vi "Main.vi"() -> ()   [LabVIEW 2019]
uses:
  UI/Channel Controls.ctl
  UI/Channel Control.ctl
  Controller/Serial Info.ctl
  UI/UI State.ctl
  UI/Update Message.ctl
  UI/Update Command.ctl
  Controller/Controller Message.ctl
  Controller/MDS Command.ctl
  UI/UI.lvlib
  Controller/Controller.lvlib
  Listener/Listener.lvlib
panel:
  in  "Listener":T1={"Port"="", "Baud Rate"=19200} {"Baud Rate" format="%.0f bps"}
  in  "Controller B":T1={"Port"="", "Baud Rate"=19200} {"Baud Rate" format="%.0f bps"}
  in  "Controller A":T1={"Port"="", "Baud Rate"=19200} {"Baud Rate" format="%.0f bps"}
  in  "Emulate":bool
  in  "Int-Ext":bool caption="Emulate"
  in  "Quit":bool
  in  "Connect":bool caption="Emulate"
  in  "Channels":T2 {"Frequency" format="%#_g MHz"; "Power" format="%#_g dBm"}
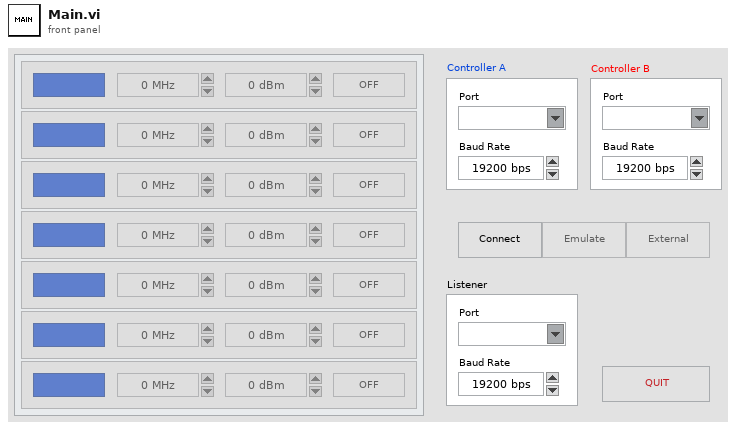
[diagram p1: front panel]
types:
  T1 = typedef "Controller.lvlib/Serial Info.ctl" = cluster{"Port":refnum<visa-resource-name>, "Baud Rate":u32}
  T2 = typedef "UI.lvlib/Channel Controls.ctl" = T3[]
  T3 = typedef "UI.lvlib/Channel Control.ctl" = cluster{"Power":dbl, "Frequency":dbl, "PLL":bool, "A/B":bool}
  T4 = typedef "UI.lvlib/UI State.ctl" = enum16{"Init", "Idle", "Update Buttons", "Connect", "Refresh Channels", "Disconnect", "Quit"}
  T5 = typedef "UI.lvlib/Main States.ctl" = cluster{"UI Queue":T6, "Controller A Queue":T7, "Controller B Queue":T7, "Listener Queue":T8}
  T6 = typedef "UI.lvlib/UI Message Queue.ctl" = refnum<queue>
  T7 = typedef "Controller.lvlib/Controller Message Queue.ctl" = refnum<queue>
  T8 = typedef "Listener.lvlib/Listener Message Queue.ctl" = refnum<queue>
  T9 = enum8{"Enabled", "Disabled", "Disabled and Grayed Out"}
  T10 = typedef "UI.lvlib/Update Message.ctl" = cluster{"Update Command":T11, "Channel":u8, "Value":variant}
  T11 = typedef "UI.lvlib/Update Command.ctl" = enum16{"Update Frequency", "Update Power", "Update Switch", "Error", "Stop"}
  T12 = typedef "Controller.lvlib/Controller Message.ctl" = cluster{"MDS Command":T13, "Channel":u8, "Value":variant}
  T13 = typedef "Controller.lvlib/MDS Command.ctl" = enum16{"Idle", "Open", "Set VMode", "Set IMode", "Get Frequency", "Set Frequency", "Get Power", "Set Power (dBm)", "Set Power (%)", "Get Switch", "Switch Channel", "Store", "Wait for Prompt", "Wait for State", "Reset", "Error", "Close", "Stop"}
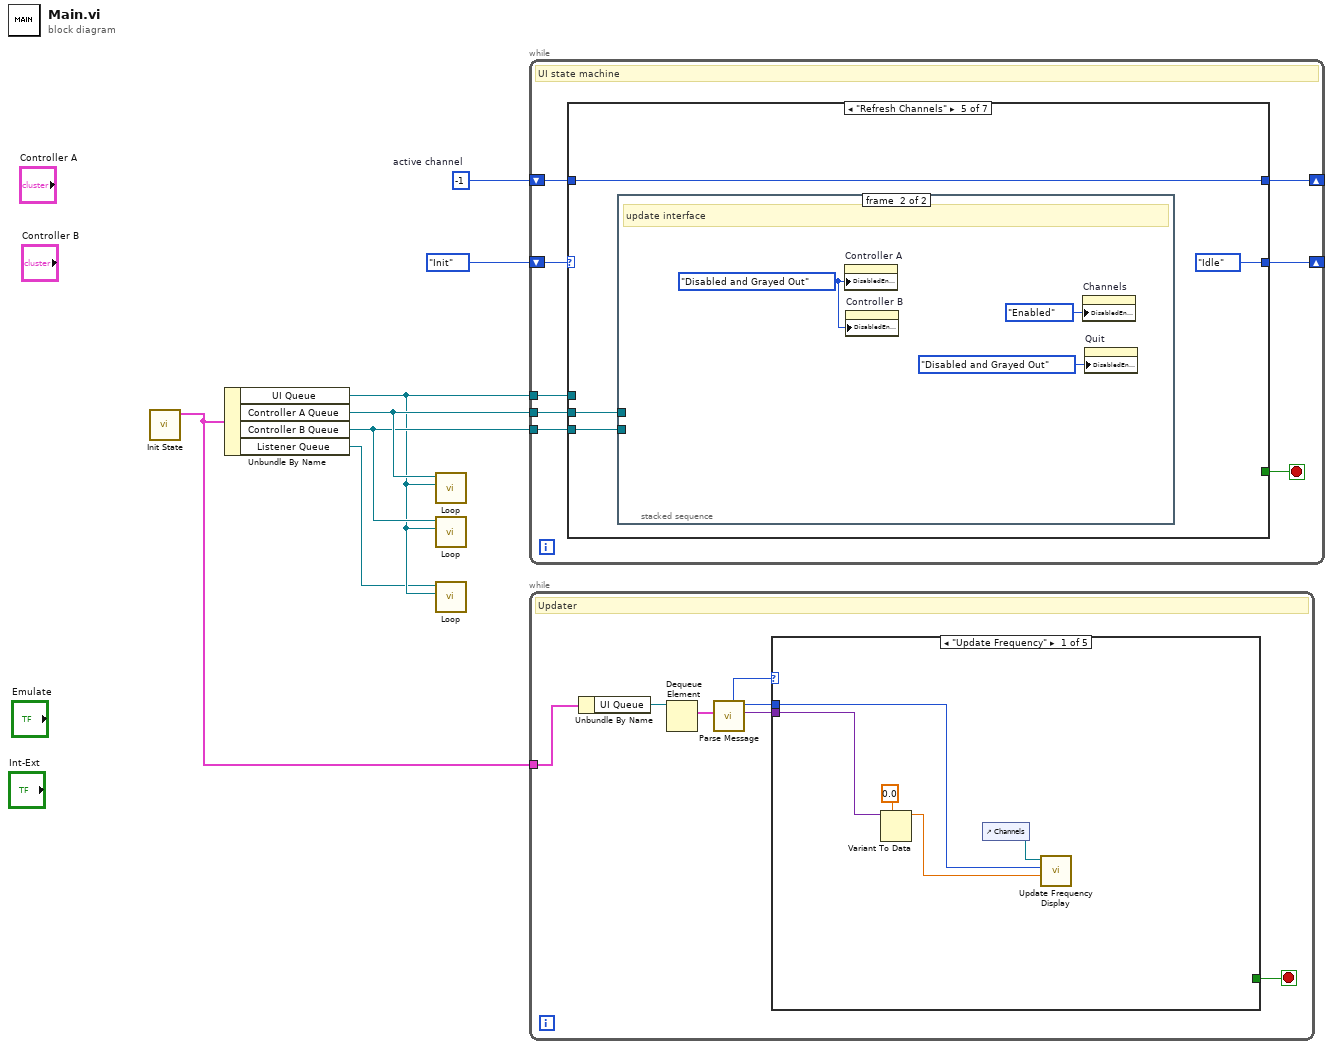
[diagram p0: block diagram]
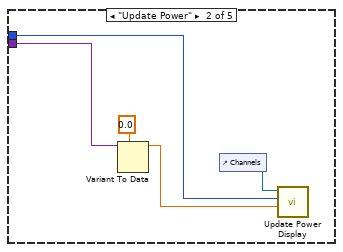
[diagram p2: hidden frame]
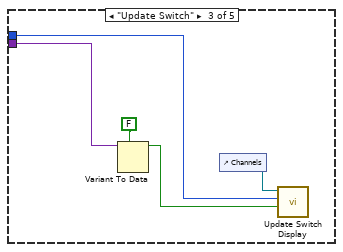
[diagram p3: hidden frame]
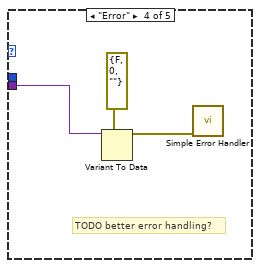
[diagram p4: hidden frame]
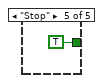
[diagram p5: hidden frame]
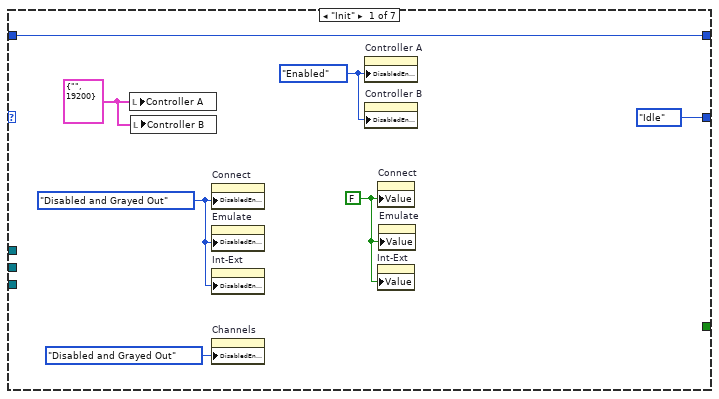
[diagram p6: hidden frame]
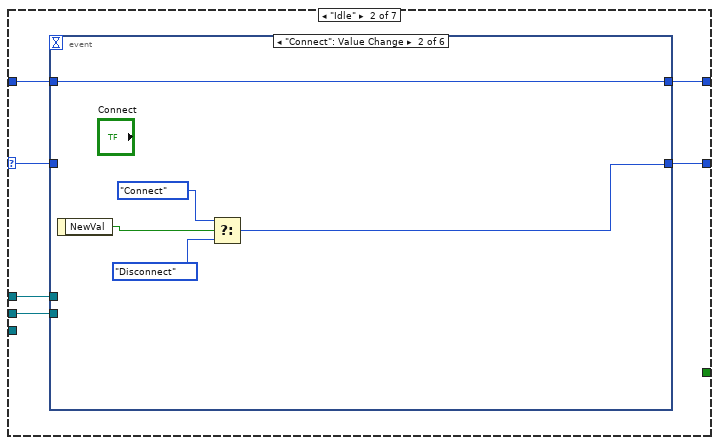
[diagram p7: hidden frame]
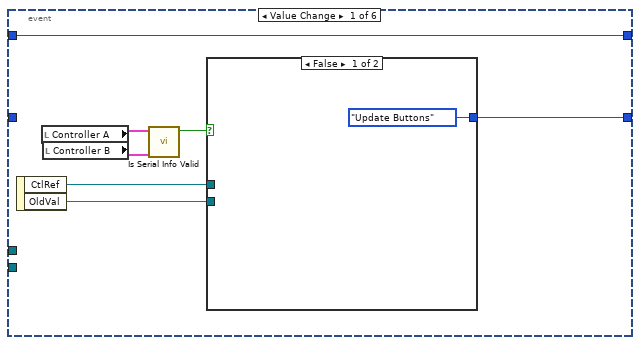
[diagram p8: hidden frame]
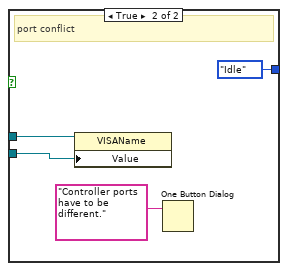
[diagram p9: hidden frame]
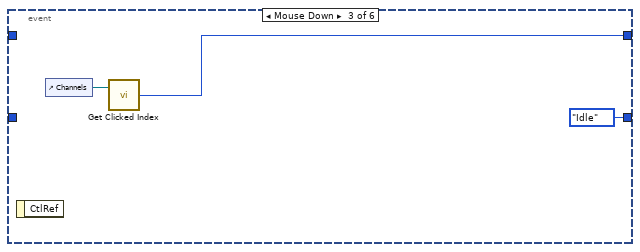
[diagram p10: hidden frame]
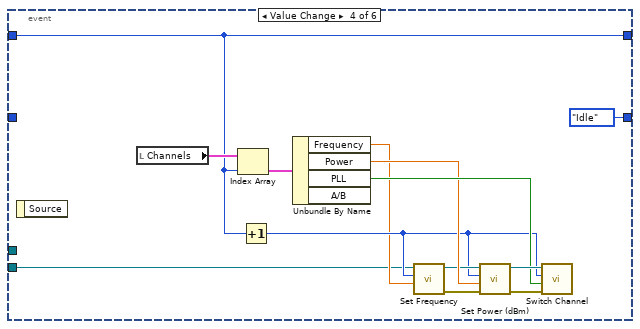
[diagram p11: hidden frame]
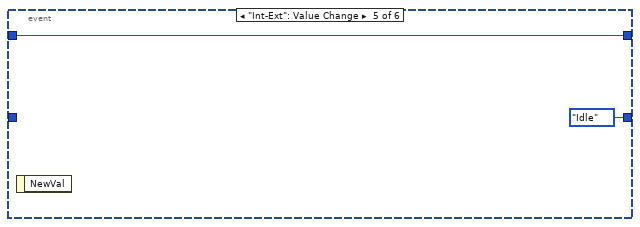
[diagram p12: hidden frame]
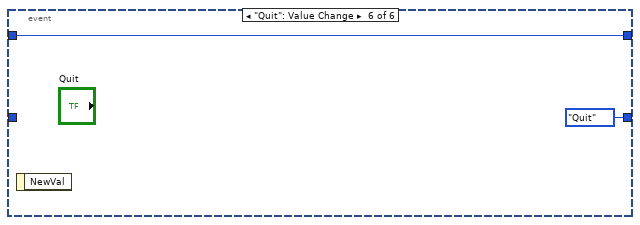
[diagram p13: hidden frame]
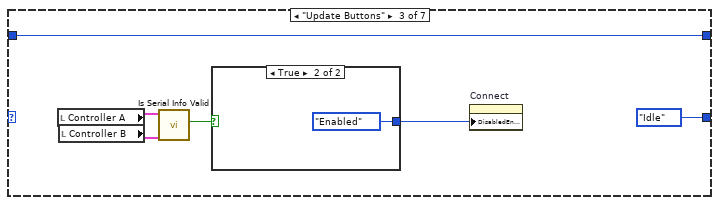
[diagram p14: hidden frame]
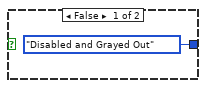
[diagram p15: hidden frame]
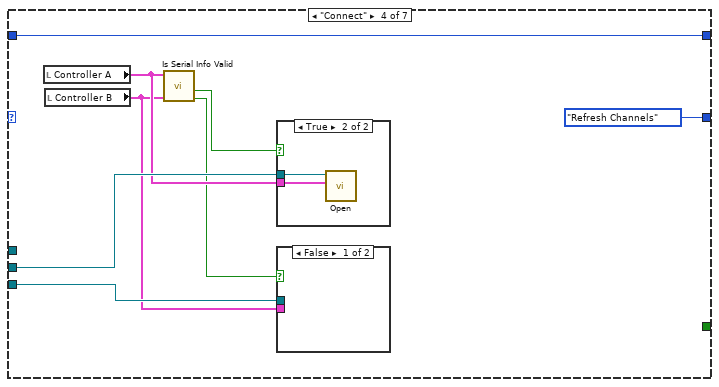
[diagram p16: hidden frame]
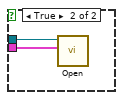
[diagram p17: hidden frame]
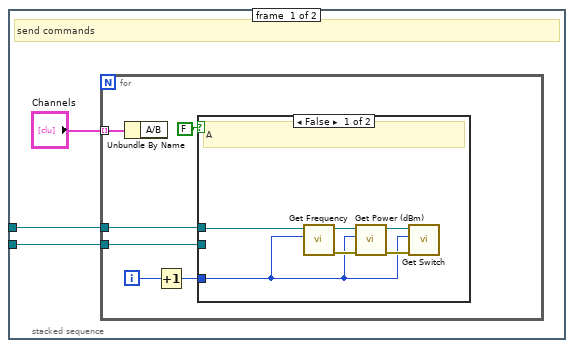
[diagram p19: hidden frame]
diagram:
  w4 = -1  # active channel
  n1 = call "Init State.vi"() -> ("Main State"=w7:T5)  [unwired: 11 in]
  n2 = Unbundle By Name(w7) -> ("UI Queue"=w2:T6, "Controller A Queue"=w5:T7, "Controller B Queue"=w3:T7, "Listener Queue"=w1:T8)
  n3 = call "Loop.vi"("UI Queue"=w2, "Controller Queue"=w5) -> ()  [unwired: 9 in, 1 out]
  n4 = call "Loop.vi"("UI Queue"=w2, "Controller Queue"=w3) -> ()  [unwired: 9 in, 1 out]
  n5 = call "Loop.vi"("UI Queue"=w2, "Listener Queue"=w1) -> ()  [unwired: 9 in, 1 out]
  n6 = while {
    tunnel: w2 -> [w15]
    shift-right: [w12] -> _
    shift-left: UI_State."Init" ("UI States") -> [w13]
    tunnel: w5 -> [w11]
    tunnel: w3 -> [w10]
    shift-right: [w9] -> _
    shift-left: w4 -> [w8]
    stop <- w14 stop-if-true
    # "UI state machine"
    n7 = case shown="\"Refresh Channels\"" w13 {
      selector: w13 -> [_ w26 _ _ _ _ _]
      tunnel: w15 -> [_ w28 _ _ _ _ w128]
      tunnel: [_ _ _ _ _ _ TRUE] -> w14
      tunnel: [UI_State."Idle" ("UI States") w27 UI_State."Idle" ("UI States") UI_State."Refresh Channels" ("UI States") UI_State."Idle" ("UI States") UI_State."Idle" ("UI States") UI_State."Quit" ("UI States")] -> w12
      tunnel: w11 -> [_ w25 _ w79 w88 w110 w126]
      tunnel: w10 -> [_ _ _ w76 w87 w109 w124]
      tunnel: [w16 w24 w66 w74 w86 w108 w125] -> w9
      tunnel: w8 -> [w16 w23 w66 w74 w86 w108 w125]
      frame "Init" {
        w17 = FALSE ("Connect")
        w18 = T9."Enabled" ("Disabled")
        w20 = T9."Disabled and Grayed Out" ("Disabled")
        w21 = T1 {"Port"="", "Baud Rate"=19200} ("Controller A")
        n8 = local write "Controller A"(w21) -> ()
        n9 = local write "Controller B"(w21) -> ()
        n10 = property on="Connect" class="Bool (strict)"("DisabledEnum"=w20) -> ()  [unwired: 2 in, 2 out]
        n11 = property on="Emulate" class="Bool (strict)"("DisabledEnum"=w20) -> ()  [unwired: 2 in, 2 out]
        n12 = property on="Int-Ext" class="Bool (strict)"("DisabledEnum"=w20) -> ()  [unwired: 2 in, 2 out]
        n13 = property on="Channels" class="Arr"("DisabledEnum"=T9."Disabled and Grayed Out" ("Disabled")) -> ()  [unwired: 2 in, 2 out]
        n14 = property on="Controller A" class="Clust (strict)"("DisabledEnum"=w18) -> ()  [unwired: 2 in, 2 out]
        n15 = property on="Controller B" class="Clust (strict)"("DisabledEnum"=w18) -> ()  [unwired: 2 in, 2 out]
        n16 = property on="Connect" class="Bool (strict)"("Value"=w17) -> ()  [unwired: 2 in, 2 out]
        n17 = property on="Int-Ext" class="Bool (strict)"("Value"=w17) -> ()  [unwired: 2 in, 2 out]
        n18 = property on="Emulate" class="Bool (strict)"("Value"=w17) -> ()  [unwired: 2 in, 2 out]
      }
      frame "Idle" {
        n19 = event shown="[1] \"Connect\": Value Change" {
          selector: _ -> [_ _ _ _ _ _]
          dyn-events: _ -> [_ _ _ _ _ _]
          timeout: _ -> [_ _ _ _ _ _]
          tunnel: w28 -> [_ _ _ _ _ _]
          tunnel: [w30 w43 UI_State."Idle" ("UI States") UI_State."Idle" ("UI States") UI_State."Idle" ("UI States") UI_State."Quit" ("UI States")] -> w27
          tunnel: w26 -> [_ _ _ _ _ _]
          tunnel: w25 -> [_ _ _ w51 _ _]
          tunnel: [w29 w41 w46 w50 w63 w64] -> w24
          tunnel: w23 -> [w29 w41 _ w50 w63 w64]
          event Value Change {
            n20 = event-data() -> ("CtlRef"=w34:refnum<vi>, "OldVal"=w33:refnum<visa-resource-name>)  [unwired: 1 in]
            n21 = local read "Controller A"() -> (w32:T1)
            n22 = local read "Controller B"() -> (w31:T1)
            n23 = call "Is Serial Info Valid.vi"("Controller B"=w31, "Controller A"=w32) -> ("Conflict?"=w35:bool)  [unwired: 6 in, 3 out]
            n24 = case shown="False" w35 {
              tunnel: w34 -> [_ w40]
              tunnel: w33 -> [_ w39]
              tunnel: [UI_State."Update Buttons" ("UI States") UI_State."Idle" ("UI States")] -> w30
              frame False {
              }
              frame True {
                # "port conflict"
                n25 = property class="VISAName"(reference=w40, "Value"=w39) -> ()  [unwired: 1 in, 2 out]
                n26 = One Button Dialog(message="Controller ports have to be different.") -> ()  [unwired: 1 in, 1 out]
              }
            }
          }
          event "Connect": Value Change {
            n27 = event-data() -> ("NewVal"=w45:bool)  [unwired: 1 in]
            n28 = Select(t=UI_State."Connect" ("UI States"), s=w45, f=UI_State."Disconnect") -> (s? t:f=w43:T4)
          }
          event Mouse Down {
            n29 = event-data() -> ()  [unwired: 1 in, 1 out]
            n30 = control-ref of="Channels"() -> (w47:refnum<vi>)
            n31 = call "Get Clicked Index.vi"("Refnum in"=w47) -> ("Index"=w46:u32)  [unwired: 1 in]
          }
          event Value Change {
            n32 = event-data() -> ()  [unwired: 1 in, 1 out]
            n33 = local read "Channels"() -> (w61:T2)
            n34 = Index Array(array=w61, index=w50) -> (element=w60:T3)
            n35 = Increment(x=w50) -> (x+1=w54:u32)
            n36 = Unbundle By Name(w60) -> ("Frequency"=w53:dbl, "Power"=w56:dbl, "PLL"=w57:bool)  [unwired: 1 out]
            n37 = call "Set Frequency.vi"("Frequency (MHz)"=w53, "Channel"=w54, "Queue in"=w51) -> ("error out"=w52:errorcluster, "Queue out"=w55:T7)  [unwired: 7 in]
            n38 = call "Set Power (dBm).vi"("error in (no error)"=w52, "Power (dBm)"=w56, "Channel"=w54, "Queue in"=w55) -> ("error out"=w58:errorcluster, "Queue out"=w59:T7)  [unwired: 6 in]
            n39 = call "Switch Channel.vi"("error in (no error)"=w58, "On/Off"=w57, "Channel"=w54, "Queue in"=w59) -> ()  [unwired: 6 in, 2 out]
          }
          event "Int-Ext": Value Change {
            n40 = event-data() -> ()  [unwired: 1 in, 1 out]
          }
          event "Quit": Value Change {
            n41 = event-data() -> ()  [unwired: 1 in, 1 out]
          }
        }
      }
      frame "Update Buttons" {
        n42 = local read "Controller A"() -> (w70:T1)
        n43 = local read "Controller B"() -> (w69:T1)
        n44 = call "Is Serial Info Valid.vi"("Controller B"=w69, "Controller A"=w70) -> ("Has Valid?"=w68:bool)  [unwired: 6 in, 3 out]
        n45 = case shown="True" w68 {
          tunnel: [T9."Disabled and Grayed Out" ("Disabled") T9."Enabled" ("Disabled")] -> w67
          frame False {
          }
          frame True {
          }
        }
        n46 = property on="Connect" class="Bool (strict)"("DisabledEnum"=w67) -> ()  [unwired: 2 in, 2 out]
      }
      frame "Connect" {
        n47 = local read "Controller A"() -> (w78:T1)
        n48 = local read "Controller B"() -> (w75:T1)
        n49 = call "Is Serial Info Valid.vi"("Controller B"=w75, "Controller A"=w78) -> ("B Valid?"=w77:bool, "A Valid?"=w80:bool)  [unwired: 6 in, 2 out]
        n50 = case shown="True" w80 {
          tunnel: w79 -> [_ w85]
          tunnel: w78 -> [_ w84]
          frame False {
          }
          frame True {
            n51 = call "Open.vi"("Serial Info"=w84, "Controller Queue in"=w85) -> ()  [unwired: 8 in, 2 out]
          }
        }
        n52 = case shown="False" w77 {
          tunnel: w76 -> [_ w83]
          tunnel: w75 -> [_ w82]
          frame False {
          }
          frame True {
            n53 = call "Open.vi"("Serial Info"=w82, "Controller Queue in"=w83) -> ()  [unwired: 8 in, 2 out]
          }
        }
      }
      frame "Refresh Channels" {
        n54 = stacked-sequence {
          tunnel: w88 -> [w91 _]
          tunnel: w87 -> [w90 _]
          frame #0 {
            # "send commands"
            n55 = for {
              tunnel: "Channels" -> [w98] mode=indexing
              tunnel: w91 -> [w96]
              tunnel: w90 -> [w95]
              i -> [w94]
              n56 = Unbundle By Name(w98) -> ()  [unwired: 1 out]
              n57 = Increment(x=w94) -> (x+1=w93:i32)
              n58 = case shown="False" FALSE {
                tunnel: w96 -> [w104 _]
                tunnel: w95 -> [_ _]
                tunnel: w93 -> [w99 _]
                frame False {
                  # "A"
                  n59 = call "Get Frequency.vi"("Channel"=w99, "Queue in"=w104) -> ("error out"=w102:errorcluster, "Queue out"=w103:T7)  [unwired: 8 in]
                  n60 = call "Get Power (dBm).vi"("error in (no error)"=w102, "Channel"=w99, "Queue in"=w103) -> ("error out"=w100:errorcluster, "Queue out"=w101:T7)  [unwired: 7 in]
                  n61 = call "Get Switch.vi"("error in (no error)"=w100, "Channel"=w99, "Queue in"=w101) -> ()  [unwired: 7 in, 2 out]
                }
                frame True {
                  # "B"
                }
              }
            }
          }
          frame #1 {
            w105 = T9."Disabled and Grayed Out" ("Disabled")
            # "update interface"
            n62 = property on="Controller A" class="Clust (strict)"("DisabledEnum"=w105) -> ()  [unwired: 2 in, 2 out]
            n63 = property on="Controller B" class="Clust (strict)"("DisabledEnum"=w105) -> ()  [unwired: 2 in, 2 out]
            n64 = property on="Channels" class="Arr"("DisabledEnum"=T9."Enabled" ("Disabled")) -> ()  [unwired: 2 in, 2 out]
            n65 = property on="Quit" class="Bool"("DisabledEnum"=T9."Disabled and Grayed Out" ("Disabled")) -> ()  [unwired: 2 in, 2 out]
          }
        }
      }
      frame "Disconnect" {
        n66 = stacked-sequence {
          tunnel: w110 -> [w116 _]
          tunnel: w109 -> [w113 _]
          frame #0 {
            # "send command"
            n67 = local read "Controller A"() -> (w115:T1)
            n68 = local read "Controller B"() -> (w112:T1)
            n69 = call "Is Serial Info Valid.vi"("Controller B"=w112, "Controller A"=w115) -> ("B Valid?"=w114:bool, "A Valid?"=w117:bool)  [unwired: 6 in, 2 out]
            n70 = case shown="True" w117 {
              tunnel: w116 -> [_ w119]
              frame False {
              }
              frame True {
                n71 = call "Close.vi"("Controller Queue in"=w119) -> ()  [unwired: 9 in, 2 out]
              }
            }
            n72 = case shown="False" w114 {
              tunnel: w113 -> [_ w118]
              frame False {
              }
              frame True {
                n73 = call "Close.vi"("Controller Queue in"=w118) -> ()  [unwired: 9 in, 2 out]
              }
            }
          }
          frame #1 {
            w120 = T9."Enabled" ("Disabled")
            # "update interface"
            n74 = property on="Controller A" class="Clust (strict)"("DisabledEnum"=w120) -> ()  [unwired: 2 in, 2 out]
            n75 = property on="Controller B" class="Clust (strict)"("DisabledEnum"=w120) -> ()  [unwired: 2 in, 2 out]
            n76 = property on="Channels" class="Arr"("DisabledEnum"=T9."Disabled and Grayed Out" ("Disabled")) -> ()  [unwired: 2 in, 2 out]
            n77 = property on="Quit" class="Bool"("DisabledEnum"=T9."Enabled" ("Disabled")) -> ()  [unwired: 2 in, 2 out]
          }
        }
      }
      frame "Quit" {
        w123 = T12 {"MDS Command"=enum."Stop", "Channel"=0, "Value"=variant} ("element")
        n78 = Enqueue Element(queue=w124, element=w123) -> ()  [unwired: 2 in, 3 out]
        n79 = Enqueue Element(queue=w126, element=w123) -> ()  [unwired: 2 in, 3 out]
        n80 = Enqueue Element(queue=w128, element=T10 {"Update Command"=enum."Stop", "Channel"=0, "Value"=variant} ("Controller Message")) -> ()  [unwired: 2 in, 3 out]
      }
    }
  }
  n81 = while {
    tunnel: w7 -> [w136]
    stop <- w131 stop-if-true
    # "Updater"
    n82 = Unbundle By Name(w136) -> ("UI Queue"=w137:T6)
    n83 = Dequeue Element(queue=w137) -> (element=w135:T10)  [unwired: 2 in, 3 out]
    n84 = call "Parse Message.vi"("Update Message"=w135) -> ("Update Command"=w134:T11, "Channel"=w133:u8, "Value"=w132:variant)  [unwired: 7 in]
    n85 = case shown="\"Update Frequency\"" w134 {
      tunnel: w133 -> [w140 w145 w150 _ _]
      tunnel: w132 -> [w142 w147 w152 w155 _]
      tunnel: [_ _ _ _ TRUE] -> w131
      frame "Update Frequency" {
        n86 = Variant To Data(type=0.0, Variant=w142) -> (data=w139:dbl)  [unwired: 1 in, 1 out]
        n87 = control-ref of="Channels"() -> (w138:refnum<vi>)
        n88 = call "Update Frequency Display.vi"("Frequency (MHz)"=w139, "Channel"=w140, "Array Refnum"=w138) -> ()  [unwired: 9 in]
      }
      frame "Update Power" {
        n89 = Variant To Data(type=0.0, Variant=w147) -> (data=w144:dbl)  [unwired: 1 in, 1 out]
        n90 = control-ref of="Channels"() -> (w143:refnum<vi>)
        n91 = call "Update Power Display.vi"("Power"=w144, "Channel"=w145, "Array Refnum"=w143) -> ()  [unwired: 9 in]
      }
      frame "Update Switch" {
        n92 = Variant To Data(type=FALSE, Variant=w152) -> (data=w149:bool)  [unwired: 1 in, 1 out]
        n93 = control-ref of="Channels"() -> (w148:refnum<vi>)
        n94 = call "Update Switch Display.vi"("On/Off"=w149, "Channel"=w150, "Array Refnum"=w148) -> ()  [unwired: 9 in]
      }
      frame "Error" {
        # "TODO better error handling?"
        n95 = Variant To Data(type=errorcluster {"status"=FALSE, "code"=0, "source"=""} ("error constant"), Variant=w155) -> (data=w153:errorcluster)  [unwired: 1 in, 1 out]
        n96 = call <vilib>:"Simple Error Handler.vi"("error in (no error)"=w153) -> ()  [unwired: 4 in, 5 out]
      }
      frame "Stop" {
      }
    }
  }
